vi "Main.vi"(7 "sweep rate, /min":dbl=0.2, 8 "sweep to:":dbl=-0.5, 9 "sweep":T6(radio)=enum."time_sweep") -> ()   [LabVIEW 2017] (continued)
                    n5481 = property on="HyperLoop" class="Bool (strict)"() -> ("Value"=w6912:bool)  [unwired: 2 in, 2 out]
                    n5482 = case shown="False" w6912 {
                      tunnel: ["_down" w6927] -> w6911
                      frame False {
                      }
                      frame True {
                        n5483 = property on="step_hyper" class="RadioBtnsControl (strict)"() -> ("Value"=w6928:T9)  [unwired: 2 in, 2 out]
                        n5484 = case shown="\"iPS_HyperLoop\"" w6928 {
                          tunnel: ["_V2400=" ("string") "_V2400=" ("string") "_Va=" ("string") "_Vb=" ("string") "_t=" ("string") "_T=" ("string") "_B" ("string")] -> w6923
                          tunnel: ["V" ("string") "V" ("string") "V" ("string") "V" ("string") _ "K" ("string") "T" ("string")] -> w6922
                          frame "2400_1_HyperLoop", Default {
                          }
                          frame "2400_2_HyperLoop" {
                          }
                          frame "2636_smua_HyperLoop" {
                          }
                          frame "2636_smub_HyperLoop" {
                          }
                          frame "time_HyperLoop" {
                          }
                          frame "iTC_HyperLoop" {
                          }
                          frame "iPS_HyperLoop" {
                          }
                        }
                        n5485 = property on="Current Hyper Value" class="DigNum (strict)"() -> ("Value"=w6925:dbl)  [unwired: 2 in, 2 out]
                        n5486 = Number To Exponential String(number=w6925) -> (E-format string=w6924:string)  [unwired: 3 in]
                        n5487 = Concatenate Strings("_down" ("string"), w6923, w6924, w6922) -> (w6927:string)
                      }
                    }
                    n5488 = Concatenate Strings(w6915, w6911) -> (w6913:string)
                    n5489 = call "AutoNamerDatExtraArtem.vi"("SweepType"=w6913, "Custom User Path"=w6916) -> ("String"=w6919:string, "Path"=w6920:path)  [unwired: 2 in]
                    n5490 = Path To String(path=w6920) -> (string=w6918:string)
                    n5491 = Concatenate Strings(w6918, "\\", w6919) -> (→"DownNameString":string)
                  }
                }
              }
              frame True {
              }
            }
          }
          frame #4 {
            n5492 = Flush Queue(queue=w6943) -> (queue out=w6942:refnum<queue>)  [unwired: 1 in, 2 out]
            n5493 = Enqueue Element(queue=w6942, element="Ramp To Limit") -> ()  [unwired: 2 in, 3 out]
          }
        }
      }
      event "Start HyperLoop", "Super Hidden": Value Change {
        n5494 = event-data() -> ()  [unwired: 1 in, 6 out]
        n5495 = stacked-sequence {
          tunnel: w6945 -> [_ _ _ w6997]
          frame #0 {
            n5496 = property on="HyperLoop Steps" class="Tbl (strict)"("Active Cell"=cluster{"Row":i32, "Column":i32} {"Row"=-2, "Column"=-2}, "Cell BG Color"=u32 16448250 ("Active Cell:Cell Background Color")) -> ()  [unwired: 2 in, 2 out]
          }
          frame #1 {
            n5497 = property on="Stop HyperLoop" class="Bool"("DisabledEnum"=T12."Enabled" ("Disabled")) -> ()  [unwired: 2 in, 2 out]
            n5498 = property on="Sweep Direction_Hyper" class="Str"("Value"="Ramp Down" ("String"), "Text.TextColor"=u32 0 ("Text.Text Colors:Text Color")) -> ()  [unwired: 2 in, 2 out]
            n5499 = property on="HyperLoop Index" class="DigNum (strict)"("Value"=0.0 ("Table Index")) -> ()  [unwired: 2 in, 2 out]
            n5500 = property on="Start HyperLoop" class="Bool"("DisabledEnum"=T12."Disabled and Grayed Out" ("Disabled")) -> ()  [unwired: 2 in, 2 out]
          }
          frame #2 {
            n5501 = property on="SuperHyper" class="Bool (strict)"() -> ("Value"=w6953:bool)  [unwired: 2 in, 2 out]
            n5502 = case shown="False" w6953 {
              frame False {
                # "Reserve two name strings for new hyperloop mapping data file:\none for up\none for down"
                n5503 = property on="Data Folder" class="Path"() -> ("Value"=w6955:path)  [unwired: 2 in, 2 out]
                n5504 = property on="MappingName" class="Str"() -> ("Value"=w6954:string)  [unwired: 2 in, 2 out]
                n5505 = stacked-sequence {
                  tunnel: w6955 -> [w6964 w6984]
                  tunnel: w6954 -> [w6963 w6983]
                  frame #0 {
                    # "Up mapping"
                    n5506 = property on="step_hyper" class="RadioBtnsControl (strict)"() -> ("Value"=w6960:T9)  [unwired: 2 in, 2 out]
                    n5507 = case shown="\"2636_smua_HyperLoop\"" w6960 {
                      tunnel: ["_V2400" ("string") "_V2400" ("string") "_Va" ("string") "_Vb" ("string") "_t" ("string") "_T" ("string") "_B" ("string")] -> w6959
                      frame "2400_1_HyperLoop", Default {
                        (unwired) "V" ("string")
                      }
                      frame "2400_2_HyperLoop" {
                        (unwired) "V" ("string")
                      }
                      frame "2636_smua_HyperLoop" {
                        (unwired) "V" ("string")
                      }
                      frame "2636_smub_HyperLoop" {
                        (unwired) "V" ("string")
                      }
                      frame "time_HyperLoop" {
                      }
                      frame "iTC_HyperLoop" {
                      }
                      frame "iPS_HyperLoop" {
                        (unwired) "T" ("string")
                      }
                    }
                    n5508 = Concatenate Strings("_HyperLoop" ("string"), w6959, "_up" ("string")) -> (w6961:string)
                    n5509 = Concatenate Strings(w6963, w6961) -> (w6962:string)
                    n5510 = call "AutoNamerDatExtraArtem.vi"("SweepType"=w6962, "Custom User Path"=w6964) -> ("String"=w6967:string, "Path"=w6968:path)  [unwired: 2 in]
                    n5511 = Path To String(path=w6968) -> (string=w6966:string)
                    n5512 = Concatenate Strings(w6966, "\\", w6967) -> (w6956:string)
                    n5513 = property on="UpNameString" class="Str"("Value"=w6956) -> ()  [unwired: 2 in, 2 out]
                  }
                  frame #1 {
                    # "Down mapping"
                    n5514 = property on="step_hyper" class="RadioBtnsControl (strict)"() -> ("Value"=w6980:T9)  [unwired: 2 in, 2 out]
                    n5515 = case shown="\"2400_2_HyperLoop\"" w6980 {
                      tunnel: ["_V2400" ("string") "_V2400" ("string") "_Va" ("string") "_Vb" ("string") "_t" ("string") "_T" ("string") "_B" ("string")] -> w6979
                      frame "2400_1_HyperLoop", Default {
                        (unwired) "V" ("string")
                      }
                      frame "2400_2_HyperLoop" {
                        (unwired) "V" ("string")
                      }
                      frame "2636_smua_HyperLoop" {
                        (unwired) "V" ("string")
                      }
                      frame "2636_smub_HyperLoop" {
                        (unwired) "V" ("string")
                      }
                      frame "time_HyperLoop" {
                      }
                      frame "iTC_HyperLoop" {
                        (unwired) "K" ("string")
                      }
                      frame "iPS_HyperLoop" {
                      }
                    }
                    n5516 = Concatenate Strings("_HyperLoop" ("string"), w6979, "_down" ("string")) -> (w6981:string)
                    n5517 = Concatenate Strings(w6983, w6981) -> (w6982:string)
                    n5518 = call "AutoNamerDatExtraArtem.vi"("SweepType"=w6982, "Custom User Path"=w6984) -> ("String"=w6987:string, "Path"=w6988:path)  [unwired: 2 in]
                    n5519 = Path To String(path=w6988) -> (string=w6986:string)
                    n5520 = Concatenate Strings(w6986, "\\", w6987) -> (w6976:string)
                    n5521 = property on="DownNameString" class="Str"("Value"=w6976) -> ()  [unwired: 2 in, 2 out]
                  }
                }
              }
              frame True {
              }
            }
          }
          frame #3 {
            n5522 = Flush Queue(queue=w6997) -> (queue out=w6996:refnum<queue>)  [unwired: 1 in, 2 out]
            n5523 = Enqueue Element(queue=w6996, element="Step to Next HyperLoop Value") -> ()  [unwired: 2 in, 3 out]
          }
        }
      }
      event "StartSuperHyper": Value Change {
        n5524 = event-data() -> ()  [unwired: 1 in, 6 out]
        n5525 = stacked-sequence {
          tunnel: w6999 -> [_ _ _ w7050]
          frame #0 {
            n5526 = property on="SuperHyper Steps" class="Tbl (strict)"("Active Cell"=cluster{"Row":i32, "Column":i32} {"Row"=-2, "Column"=-2}, "Cell BG Color"=u32 16448250 ("Active Cell:Cell Background Color")) -> ()  [unwired: 2 in, 2 out]
          }
          frame #1 {
            n5527 = property on="Stop SuperHyper" class="Bool"("DisabledEnum"=T12."Enabled" ("Disabled")) -> ()  [unwired: 2 in, 2 out]
            n5528 = property on="SuperHyper_Index" class="DigNum (strict)"("Value"=0.0 ("Table Index")) -> ()  [unwired: 2 in, 2 out]
            n5529 = property on="StartSuperHyper" class="Bool"("DisabledEnum"=T12."Disabled and Grayed Out" ("Disabled")) -> ()  [unwired: 2 in, 2 out]
            n5530 = property on="Sweep Direction3" class="Str"("Value"="Ramp Down" ("String"), "Text.TextColor"=u32 0 ("Text.Text Colors:Text Color")) -> ()  [unwired: 2 in, 2 out]
          }
          frame #2 {
            # "Reserve two name strings for new hyperloop mapping data file:\none for up\none for down"
            n5531 = property on="Data Folder" class="Path"() -> ("Value"=w7008:path)  [unwired: 2 in, 2 out]
            n5532 = property on="MappingName" class="Str"() -> ("Value"=w7007:string)  [unwired: 2 in, 2 out]
            n5533 = stacked-sequence {
              tunnel: w7008 -> [w7017 w7037]
              tunnel: w7007 -> [w7016 w7036]
              frame #0 {
                # "Up mapping"
                n5534 = property on="Step_SuperHyper" class="RadioBtnsControl (strict)"() -> ("Value"=w7009:T10)  [unwired: 2 in, 2 out]
                n5535 = case shown="\"2400_1_SuperHyper\", Default" w7009 {
                  tunnel: ["_V2400" ("string") "_V2400" ("string") "_Va" ("string") "_Vb" ("string") "_t" ("string") "_T" ("string") "_B" ("string")] -> w7013
                  frame "2400_1_SuperHyper", Default {
                    (unwired) "V" ("string")
                  }
                  frame "2400_2_SuperHyper" {
                    (unwired) "V" ("string")
                  }
                  frame "2636_smua_SuperHyper" {
                    (unwired) "V" ("string")
                  }
                  frame "2636_smub_SuperHyper" {
                    (unwired) "V" ("string")
                  }
                  frame "time_SuperHyper" {
                  }
                  frame "iTC_SuperHyper" {
                  }
                  frame "iPS_SuperHyper" {
                    (unwired) "T" ("string")
                  }
                }
                n5536 = Concatenate Strings("_SuperHyper" ("string"), w7013, "_up" ("string")) -> (w7014:string)
                n5537 = Concatenate Strings(w7016, w7014) -> (w7015:string)
                n5538 = call "AutoNamerDatExtraArtem.vi"("SweepType"=w7015, "Custom User Path"=w7017) -> ("String"=w7020:string, "Path"=w7021:path)  [unwired: 2 in]
                n5539 = Path To String(path=w7021) -> (string=w7019:string)
                n5540 = Concatenate Strings(w7019, "\\", w7020) -> (w7010:string)
                n5541 = property on="UpNameString" class="Str"("Value"=w7010) -> ()  [unwired: 2 in, 2 out]
              }
              frame #1 {
                # "Down mapping"
                n5542 = property on="Step_SuperHyper" class="RadioBtnsControl (strict)"() -> ("Value"=w7029:T10)  [unwired: 2 in, 2 out]
                n5543 = case shown="\"2400_2_SuperHyper\"" w7029 {
                  tunnel: ["_V2400" ("string") "_V2400" ("string") "_Va" ("string") "_Vb" ("string") "_t" ("string") "_T" ("string") "_B" ("string")] -> w7033
                  frame "2400_1_SuperHyper", Default {
                    (unwired) "V" ("string")
                  }
                  frame "2400_2_SuperHyper" {
                    (unwired) "V" ("string")
                  }
                  frame "2636_smua_SuperHyper" {
                    (unwired) "V" ("string")
                  }
                  frame "2636_smub_SuperHyper" {
                    (unwired) "V" ("string")
                  }
                  frame "time_SuperHyper" {
                  }
                  frame "iTC_SuperHyper" {
                    (unwired) "K" ("string")
                  }
                  frame "iPS_SuperHyper" {
                  }
                }
                n5544 = Concatenate Strings("_SuperHyper" ("string"), w7033, "_down" ("string")) -> (w7034:string)
                n5545 = Concatenate Strings(w7036, w7034) -> (w7035:string)
                n5546 = call "AutoNamerDatExtraArtem.vi"("SweepType"=w7035, "Custom User Path"=w7037) -> ("String"=w7040:string, "Path"=w7041:path)  [unwired: 2 in]
                n5547 = Path To String(path=w7041) -> (string=w7039:string)
                n5548 = Concatenate Strings(w7039, "\\", w7040) -> (w7030:string)
                n5549 = property on="DownNameString" class="Str"("Value"=w7030) -> ()  [unwired: 2 in, 2 out]
              }
            }
          }
          frame #3 {
            n5550 = Flush Queue(queue=w7050) -> (queue out=w7049:refnum<queue>)  [unwired: 1 in, 2 out]
            n5551 = Enqueue Element(queue=w7049, element="Step to Next SuperHyper Value") -> ()  [unwired: 2 in, 3 out]
          }
        }
      }
      event "Monitor": Value Change {
        n5552 = event-data() -> ()  [unwired: 1 in, 6 out]
        n5553 = case shown="True" "Monitor" {
          frame True {
            w7053 = TRUE ("Visible")
            n5554 = property on="Figure_axis" class="Arr (strict)"("Visible"=w7053) -> ()  [unwired: 2 in, 2 out]
            n5555 = property on="data" class="Arr (strict)"("Visible"=w7053) -> ()  [unwired: 2 in, 2 out]
            n5556 = property on="formula_variables" class="Arr (strict)"("Visible"=w7053) -> ()  [unwired: 2 in, 2 out]
          }
          frame False {
            w7054 = FALSE ("Visible")
            n5557 = property on="Figure_axis" class="Arr (strict)"("Visible"=w7054) -> ()  [unwired: 2 in, 2 out]
            n5558 = property on="formula_variables" class="Arr (strict)"("Visible"=w7054) -> ()  [unwired: 2 in, 2 out]
            n5559 = property on="data" class="Arr (strict)"("Visible"=w7054) -> ()  [unwired: 2 in, 2 out]
          }
        }
      }
      event "TempCtrl", "MagnetCtrl": Value Change {
        n5560 = event-data() -> ("CtlRef"=w7067:refnum<vi>)  [unwired: 1 in, 5 out]
        n5561 = property class="Bool"(reference=w7067) -> ("Label.Text"=w7066:string)  [unwired: 1 in, 2 out]
        n5562 = case shown="\"MagnetCtrl\"" w7066 {
          tunnel: w7057 -> [w7074 w7077]
          tunnel: [w7073 w7076] -> w7065
          tunnel: [w7072 w7075] -> w7061
          frame "TempCtrl", Default {
            n5563 = property on="iTC_addr_sweep" class="VISAName"() -> ("Value"=w7072:refnum<visa-resource-name>)  [unwired: 2 in, 2 out]
            n5564 = Unbundle(w7074) -> ("vi reference"=w7073:refnum<vi>)  [unwired: 1 out]
          }
          frame "MagnetCtrl" {
            n5565 = Unbundle(w7077) -> ("vi reference"=w7076:refnum<vi>)  [unwired: 1 out]
            n5566 = property on="iPS_addr_sweep" class="VISAName"() -> ("Value"=w7075:refnum<visa-resource-name>)  [unwired: 2 in, 2 out]
          }
        }
        n5567 = invoke class="VI" method="FP.Open"(reference=w7065, "Activate"=TRUE ("Activate?")) -> (reference out=w7063:refnum<vi>)  [unwired: 3 in, 4 out]
        n5568 = invoke class="VI" method="Ctrl Val.Set"(reference=w7063, "Control Name"="VISA resource name", "Value"=w7061) -> (reference out=w7060:refnum<vi>)  [unwired: 2 in, 4 out]
        n5569 = property class="VI"(reference=w7060) -> (reference out=w7058:refnum<vi>, "Exec.State"=w7059:T23)  [unwired: 1 in, 1 out]
        n5570 = case shown="\"Idle\"" w7059 {
          tunnel: w7058 -> [w7068 w7071]
          tunnel: [w7068 w7069] -> w7056
          frame "Bad", Default {
          }
          frame "Idle" {
            n5571 = invoke class="VI" method="Run VI"(reference=w7071, "Wait until done"=FALSE ("Wait Until Done")) -> (reference out=w7069:refnum<vi>)  [unwired: 3 in, 4 out]
          }
        }
        n5572 = property class="VI"(reference=w7056, "Front Panel.IsFrontmost"=TRUE ("Front Panel Window:Is Frontmost")) -> ()  [unwired: 1 in, 2 out]
      }
      event "Lockin_Setup", "Cytec_Switch": Value Change {
        n5573 = event-data() -> ("CtlRef"=w7084:refnum<vi>)  [unwired: 1 in, 5 out]
        n5574 = property class="Bool"(reference=w7084) -> ("Label.Text"=w7083:string)  [unwired: 1 in, 2 out]
        n5575 = case shown="\"Cytec_Switch\", Default" w7083 {
          tunnel: w7082 -> [w7089 w7091]
          tunnel: [w7088 w7090] -> w7081
          frame "Cytec_Switch", Default {
            n5576 = Unbundle(w7089) -> ("vi reference"=w7088:refnum<vi>)  [unwired: 1 out]
          }
          frame "Lockin_Setup" {
            n5577 = Unbundle(w7091) -> ("vi reference"=w7090:refnum<vi>)  [unwired: 1 out]
          }
        }
        n5578 = invoke class="VI" method="FP.Open"(reference=w7081, "Activate"=TRUE ("Activate?")) -> (reference out=w7079:refnum<vi>)  [unwired: 3 in, 4 out]
        n5579 = property class="VI"(reference=w7079) -> (reference out=w7078:refnum<vi>, "Exec.State"=w7080:T23)  [unwired: 1 in, 1 out]
        n5580 = case shown="\"Idle\"" w7080 {
          tunnel: w7078 -> [_ w7086]
          frame "Bad", Default {
          }
          frame "Idle" {
            n5581 = invoke class="VI" method="Run VI"(reference=w7086, "Wait until done"=FALSE ("Wait Until Done")) -> ()  [unwired: 3 in, 5 out]
          }
        }
      }
    }
  }
  n5582 = Release Queue(queue=w4) -> ()  [unwired: 2 in, 3 out]
